vi "Set Column Widths.vi"(8 "error in":errorcluster, 9 "Widths":i32[](array[numeric]), 10 "Cols":i32[](array[numeric]), 11 "Sourcegrid in":refnum<class "SourceGrid.lvclass">) -> (0 "error out":errorcluster, 3 "Sourcegrid out":refnum<class "SourceGrid.lvclass">)   [LabVIEW 2023, in "SourceGrid.lvlib" / "SourceGrid.lvclass"]
uses:
  SourceGrid.lvclass
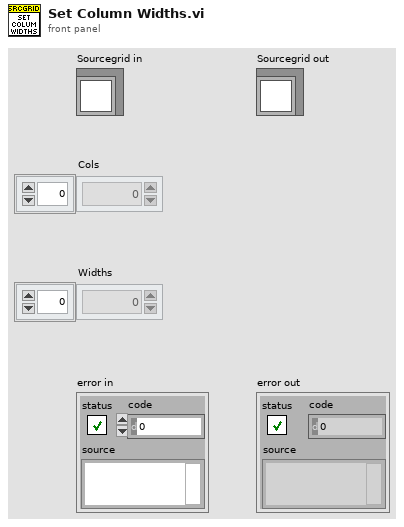
[diagram p1: front panel]
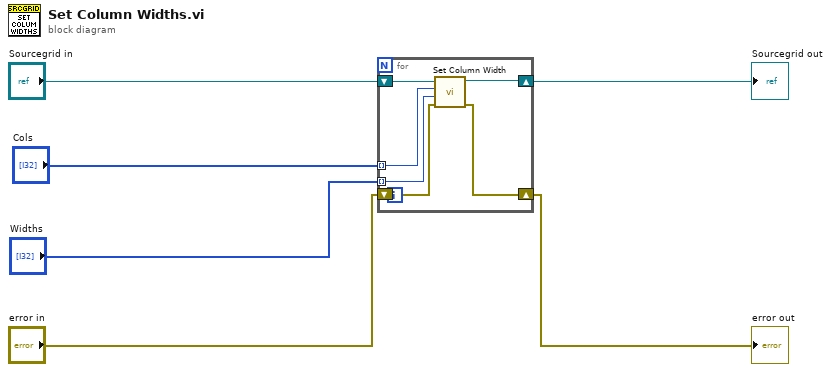
[diagram p0: block diagram]
diagram:
  n1 = for {
    tunnel: "Cols" -> [w9] mode=indexing
    tunnel: "Widths" -> [w8] mode=indexing
    shift-right: [w7] -> w1
    shift-left: "Sourcegrid in" -> [w12]
    shift-right: [w10] -> w2
    shift-left: "error in" -> [w11]
    n2 = call "Set Column Width.vi"("error in"=w11, "Width"=w8, "Column"=w9, "Sourcegrid in"=w12) -> ("error out"=w10:errorcluster, "Sourcegrid out"=w7:refnum<class "SourceGrid.lvclass">)  [unwired: 6 in]
  }
  "error out" <- w2
  "Sourcegrid out" <- w1
